vi "fill_elements_by_name.vi"(5 "little-endian arrays (T)":bool=TRUE, 8 "error in (no error)":errorcluster, 10 "arrayOfElements":T1[](array[typedef]), 11 "dataType in":variant) -> (0 "error out":errorcluster, 3 "dataType out":variant)   [LabVIEW 2015, in "BSON_convertors_Library.lvlib"]
uses:
  BSON_convertors_Library.lvlib
  typedefs/BSONelement.ctl
  typedefs/dataType.ctl
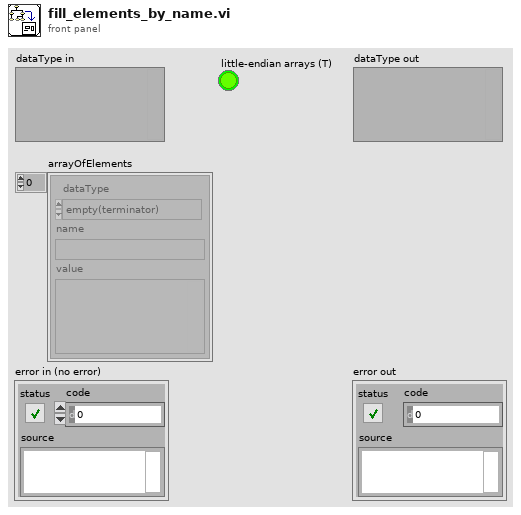
[diagram p1: front panel]
types:
  T1 = typedef "BSON_convertors_Library.lvlib/BSONelement.ctl" = cluster{"dataType":T2, "name":string, "value":variant}
  T2 = typedef "BSON_convertors_Library.lvlib/dataType.ctl" = enum8{"empty(terminator)", "double", "string", "document", "array", "binary", "Deprecated(Undefined)", "ObjectId", "boolean", "UTC datetime", "Null value", "cstring", "Deprecated(DBPointer)", "JavaScript", "Deprecated(Symbol)", "code_w_s", "int32", "uint64", "int64", "ext (decimal128)", "Min key", "Max key"}
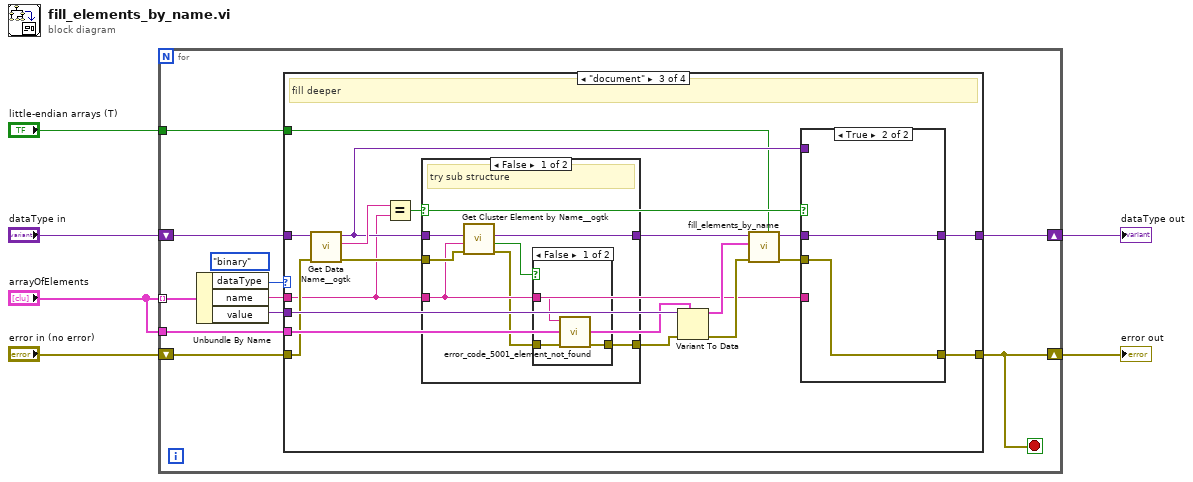
[diagram p0: block diagram]
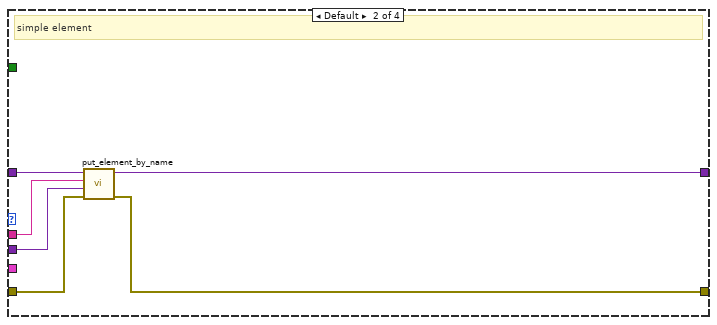
[diagram p3: hidden frame]
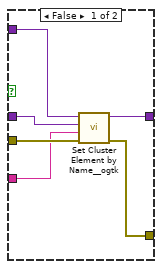
[diagram p4: hidden frame]
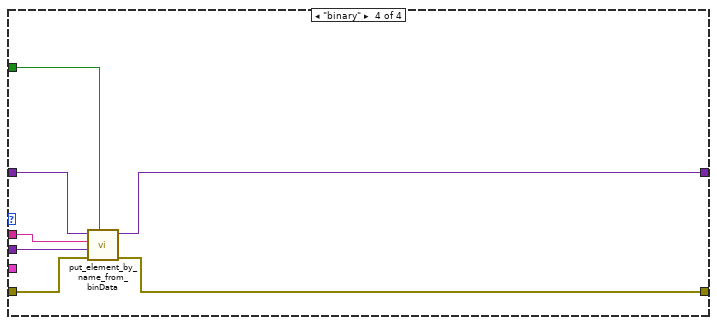
[diagram p7: hidden frame]
diagram:
  n1 = for {
    tunnel: "arrayOfElements" -> [w16] mode=indexing
    shift-right: [w9] -> w4
    shift-left: "error in (no error)" -> [w10]
    shift-right: [w13] -> w5
    shift-left: "dataType in" -> [w14]
    tunnel: "arrayOfElements" -> [w8]
    tunnel: "little-endian arrays (T)" -> [w7]
    stop <- w9 stop-if-true
    (unwired) dataType."binary" ("dataType")
    n2 = Unbundle By Name(w16) -> ("dataType"=w15:T2, "name"=w12:string, "value"=w11:variant)
    n3 = case shown="\"document\"" w15 {
      tunnel: w14 -> [w18 w24 w40 w68]
      tunnel: [w18 w23 w29 w67] -> w13
      tunnel: w12 -> [_ w19 w26 w66]
      tunnel: w11 -> [_ w22 w42 w70]
      tunnel: w10 -> [w17 w21 w38 w69]
      tunnel: [w17 w20 w27 w65] -> w9
      tunnel: w8 -> [_ _ w41 _]
      tunnel: w7 -> [_ _ w25 w64]
      frame "empty(terminator)" {
      }
      frame Default {
        # "simple element"
        n4 = call "put_element_by_name.vi"("error in (no error)"=w21, "value"=w22, "name"=w19, "dataType in"=w24) -> ("error out"=w20:errorcluster, "data out"=w23:variant)  [unwired: 6 in]
      }
      frame "document" {
        # "fill deeper"
        n5 = call <userlib>:"Get Data Name__ogtk.vi"("error in (no error)"=w38, "Data"=w40) -> ("error out"=w34:errorcluster, "Data Name"=w39:string, "Data dup"=w28:variant)  [unwired: 7 in]
        n6 = Equal?(x=w39, y=w26) -> (x = y?=w32:bool)
        n7 = case shown="False" w32 {
          tunnel: [w56 w63] -> w35
          tunnel: w28 -> [w57 w63]
          tunnel: w26 -> [w51 _]
          tunnel: w34 -> [w55 w62]
          tunnel: [w53 w62] -> w33
          frame False {
            # "try sub structure"
            n8 = call <userlib>:"Get Cluster Element by Name__ogtk.vi"("error in (no error)"=w55, "Element Name"=w51, "Cluster"=w57) -> ("error out"=w54:errorcluster, "found?"=w52:bool, "VElement"=w56:variant)  [unwired: 6 in]
            n9 = case shown="False" w52 {
              tunnel: w54 -> [w60 w61]
              tunnel: [w59 w61] -> w53
              tunnel: w51 -> [w58 _]
              frame False {
                n10 = call "error_code_5001_element_not_found.vi"("error in (no error)"=w60, "name"=w58) -> ("error out"=w59:errorcluster)  [unwired: 9 in]
              }
              frame True {
              }
            }
          }
          frame True {
            # "fill root"
          }
        }
        n11 = Variant To Data(error in=w33, type=w41, Variant=w42) -> (data=w37:T1[], error out=w36:errorcluster)
        n12 = call "fill_elements_by_name.vi"("little-endian arrays (T)"=w25, "error in (no error)"=w36, "arrayOfElements"=w37, "dataType in"=w35) -> ("error out"=w30:errorcluster, "dataType out"=w31:variant)  [unwired: 6 in]
        n13 = case shown="True" w32 {
          tunnel: w31 -> [w46 w50]
          tunnel: w30 -> [w45 w49]
          tunnel: [w47 w50] -> w29
          tunnel: w28 -> [w48 _]
          tunnel: w26 -> [w44 _]
          tunnel: [w43 w49] -> w27
          frame False {
            n14 = call <userlib>:"Set Cluster Element by Name__ogtk.vi"("error in (no error)"=w45, "Element Name (\"\": New Element Data Name)"=w44, "New Element Value"=w46, "Cluster"=w48) -> ("error out"=w43:errorcluster, "VCluster out"=w47:variant)  [unwired: 5 in, 1 out]
          }
          frame True {
          }
        }
      }
      frame "binary" {
        n15 = call "put_element_by_name_from_binData.vi"("little-endian?"=w64, "error in (no error)"=w69, "value"=w70, "name"=w66, "dataType in"=w68) -> ("error out"=w65:errorcluster, "data out"=w67:variant)  [unwired: 5 in]
      }
    }
  }
  "dataType out" <- w5
  "error out" <- w4
